vi "Read Motor Speed.vi"(6 "error in":errorcluster, 8 "MaxRead":i32, 9 "Channel in":u16) -> (0 "error out":errorcluster, 1 "Messages":T1(array[cluster]), 2 "Pass":bool, 3 "Channel out":u16, 4 "FloatNumber":sgl)   [LabVIEW 2023]
uses:
  c60d9e91-3b79-4ba4-9146-ee67ae1b5e7d.vi
  Communication/PCAN2023/PCAN API.lvlib
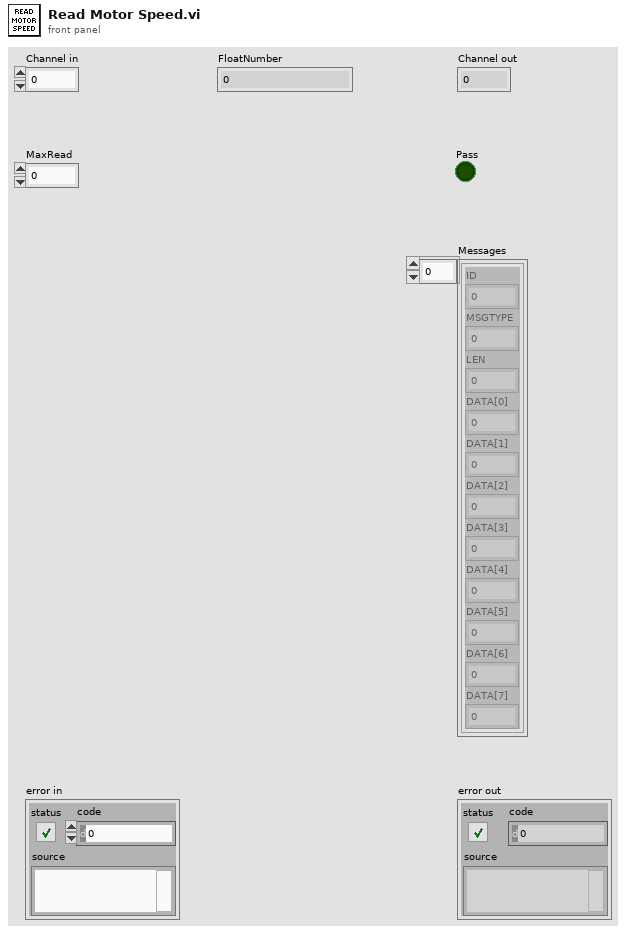
[diagram p1: front panel]
types:
  T1 = cluster{"ID":u32, "MSGTYPE":u8, "LEN":u8, "DATA[0]":u8, "DATA[1]":u8, "DATA[2]":u8, "DATA[3]":u8, "DATA[4]":u8, "DATA[5]":u8, "DATA[6]":u8, "DATA[7]":u8}[]
  T2 = cluster{"ID":u32, "MSGTYPE":u8, "LEN":u8, "DATA[0]":u8, "DATA[1]":u8, "DATA[2]":u8, "DATA[3]":u8, "DATA[4]":u8, "DATA[5]":u8, "DATA[6]":u8, "DATA[7]":u8}
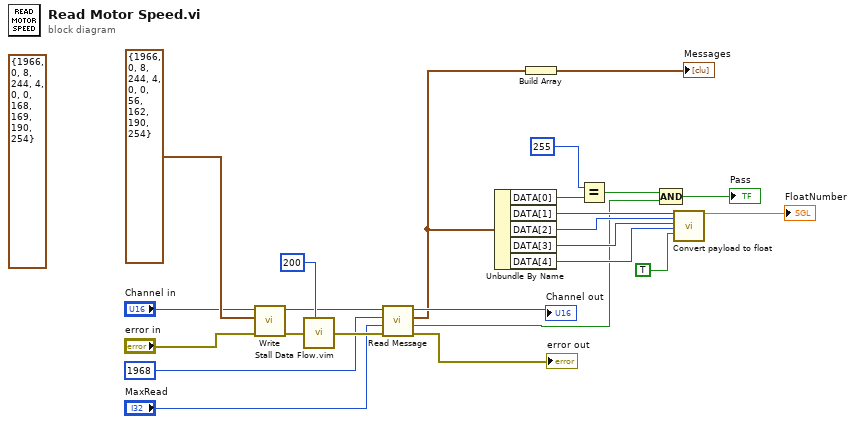
[diagram p0: block diagram]
diagram:
  (unwired) T2 {"ID"=1966, "MSGTYPE"=0, "LEN"=8, "DATA[0]"=244, "DATA[1]"=4, "DATA[2]"=0, "DATA[3]"=0, "DATA[4]"=168, "DATA[5]"=169, "DATA[6]"=190, "DATA[7]"=254} ("MessageBuffer")
  n1 = call "Write.vi"("error in"="error in", "MessageBuffer"=T2 {"ID"=1966, "MSGTYPE"=0, "LEN"=8, "DATA[0]"=244, "DATA[1]"=4, "DATA[2]"=0, "DATA[3]"=0, "DATA[4]"=56, "DATA[5]"=162, "DATA[6]"=190, "DATA[7]"=254}, "Channel"="Channel in") -> ("error out"=w23:errorcluster, "Channel out"=w8:u16)  [unwired: 5 in, 2 out]
  n2 = call "Stall Data Flow.vim"("value in"=w23, "milliseconds to wait"=u32 200) -> ("value out"=w6:errorcluster)  [unwired: 1 out]
  n3 = call "Read Message.vi"("error in"=w6, "MaxRead"="MaxRead", "ID"=u32 1968, "Channel in"=w8) -> ("error out"=→"error out":errorcluster, "Passed"=w4:bool, "Last Message"=w1:T2, "Channel out"=→"Channel out":u16)  [unwired: 3 in, 1 out]
  n4 = Unbundle By Name(w1) -> ("DATA[0]"=w20:u8, "DATA[1]"=w14:u8, "DATA[2]"=w13:u8, "DATA[3]"=w12:u8, "DATA[4]"=w11:u8)
  n5 = Build Array(w1) -> (→"Messages":T1)
  n6 = Equal?(x=u8 255, y=w20) -> (x = y?=w18:bool)
  n7 = Compound Arithmetic op=AND(w18, w4) -> (→"Pass":bool)
  n8 = call "Convert payload to float.vi"("Byte1"=w14, "Byte2"=w13, "Byte3"=w12, "Byte4"=w11, "Invert"=TRUE) -> ("FloatNumber"=→"FloatNumber":sgl)  [unwired: 14 in]
